vi "TKPS252XG Initialize24.vi"(2 "error in (no error)":errorcluster, 3 "reset":bool=TRUE, 4 "ID query":bool=TRUE, 5 "VISA session (for class)":refnum<visa-resource-name>="GPIB0::8::INSTR") -> (0 "error out":errorcluster, 1 "VISA session":refnum<visa-resource-name>)   [LabVIEW 2024]
doc: "This VI loads the addressing information for the instrument and allows the user to reset the instrument by setting the front panel Reset control and checking the instrument ID by setting the front panel ID Query control.\n\nYou must run this VI before using any of the instrument driver VIs for this instrument."
panel:
  # "yes\nno"
  # "yes\nno"
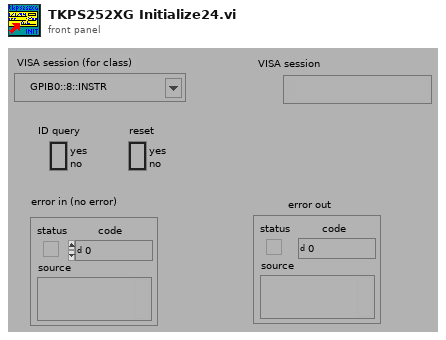
[diagram p1: front panel]
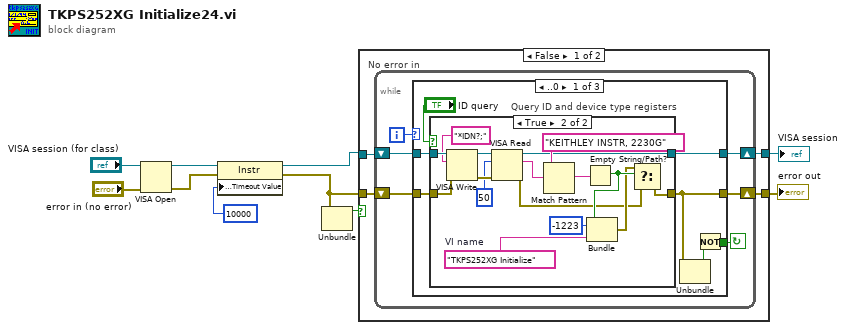
[diagram p0: block diagram]
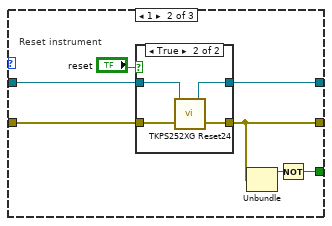
[diagram p3: hidden frame]
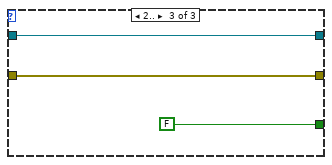
[diagram p5: hidden frame]
diagram:
  n1 = VISA Open(error in (no error)="error in (no error)", VISA resource name="VISA session (for class)") -> (VISA resource name=w1:refnum<visa-resource-name>, error out=w2:errorcluster)  [unwired: 3 in]
  n2 = property class="Instr"(reference=w1, error in=w2, "General Settings:Timeout Value"=u32 10000 ("Tmo Value")) -> (reference out=w4:refnum<visa-resource-name>, error out=w3:errorcluster)
  n3 = Unbundle(w3) -> ("status"=w10:bool)  [unwired: 2 out]
  n4 = case shown="False" w10 {
    tunnel: w3 -> [w14 w63]
    tunnel: [w13 w63] -> w9
    tunnel: [w12 w62] -> w8
    tunnel: w4 -> [w11 w62]
    frame False {
      # "No error in"
      n5 = while {
        shift-left: w11 -> [w16]
        shift-right: [w17] -> w12
        shift-left: w14 -> [w20]
        shift-right: [w19] -> w13
        i -> [w18]
        stop <- w15 continue-if-true
        n6 = case shown="..0" w18 {
          tunnel: w20 -> [w27 w52 w60]
          tunnel: [w23 w48 w60] -> w19
          tunnel: [w25 w49 w59] -> w17
          tunnel: w16 -> [w26 w50 w59]
          tunnel: [w21 w46 FALSE] -> w15
          frame ..0 {
            # "Query ID and device type registers"
            n7 = case shown="True" "ID query" {
              tunnel: [w29 w32] -> w23
              tunnel: w27 -> [w29 w43]
              tunnel: [w28 w35] -> w25
              tunnel: w26 -> [w28 w44]
              frame False {
              }
              frame True {
                w30 = "TKPS252XG Initialize"  # VI name
                n8 = VISA Write(VISA resource name=w44, write buffer="*IDN?;", error in (no error)=w43) -> (VISA resource name out=w37:refnum<visa-resource-name>, error out=w41:errorcluster)  [unwired: 1 out]
                n9 = VISA Read(VISA resource name=w37, byte count=50, error in (no error)=w41) -> (VISA resource name out=w35:refnum<visa-resource-name>, read buffer=w40:string, error out=w31:errorcluster)  [unwired: 1 out]
                n10 = Match Pattern(string=w40, regular expression="KEITHLEY INSTR, 2230G") -> (match substring=w38:string)  [unwired: 1 in, 3 out]
                n11 = Empty String/Path?(string/path=w38) -> (empty?=w34:bool)
                n12 = Bundle(w34, -1223, "VI name"=w30) -> (w33:cluster{bool, i32, "VI name":string})  [unwired: 1 in]
                n13 = Select(t=w33, s=w34, f=w31) -> (s? t:f=w32:errorcluster)
              }
            }
            n14 = Unbundle(w23) -> ("status"=w22:bool)  [unwired: 2 out]
            n15 = Not(x=w22) -> (.not. x?=w21:bool)
          }
          frame 1 {
            # "Reset instrument"
            n16 = case shown="True" "reset" {
              tunnel: w52 -> [w54 w58]
              tunnel: [w54 w56] -> w48
              tunnel: w50 -> [w53 w57]
              tunnel: [w53 w55] -> w49
              frame False {
              }
              frame True {
                n17 = call "TKPS252XG Reset24.vi"("error in (no error)"=w58, "VISA session"=w57) -> ("error out"=w56:errorcluster, "dup VISA session"=w55:refnum<visa-resource-name>)
              }
            }
            n18 = Unbundle(w48) -> ("status"=w47:bool)  [unwired: 2 out]
            n19 = Not(x=w47) -> (.not. x?=w46:bool)
          }
          frame 2.. {
          }
        }
      }
    }
    frame True {
      # "Error"
    }
  }
  "VISA session" <- w8
  "error out" <- w9
